vi "FitData.vi"(4 "Fit?":bool=TRUE, 6 "Fmax":dbl format="%#_13g", 7 "Fmin":dbl format="%#_13g", 8 "Yarray":dbl[](array[numeric])) -> (0 "Peak Area (mV-MHz)":dbl=0.0044393014138011675 format="%#_3g", 1 "Center Freq (MHz)":dbl=224.7917277288786, 2 "Amplitude (V)":dbl=0.25549081559976244 format="%#_3g", 3 "NMR Graph + Fit":cluster{cluster{dbl, "Numeric":dbl}[]}[](graph), 5 "# Data points":i32)   [LabVIEW 2018]
uses:
  <vilib>/Analysis/NI_AALPro.lvlib
panel:
  out "Numeric 3":i32
  out "Numeric 2":i32
  out "Yarray 2":dbl[](array[numeric])=[0.01394901666666204, 0.014369016666664246, 0.014784816666666256, 0.015196416666656568, 0.01560381666665861, 0.016007016666660615, 0.015406016666662567, 0.014800816666664496, 0.015191416666666374, 0.015577816666657293, 0.014960016666659214, 0.01533801666666109, 0.014711816666662929, 0.015081416666664724, 0.014446816666666487, 0.014808016666658, 0.014165016666659796, 0.014517816666661555, 0.01386641666666327, 0.014210816666664947, 0.014551016666666583, 0.013887016666658689, 0.013218816666660367, 0.013546416666662002, 0.012869816666663605, 0.013189016666665158, 0.012504016666666673, 0.01181481666665938, 0.01112141666666093, 0.010423816666662443, 0.01072201666666392, 0.011016016666665358, 0.01130581666666675, 0.010591416666660046, 0.009872816666661479, 0.010150016666662872, 0.010423016666664228, 0.010691816666665542, 0.009956416666666822, 0.009216816666660708, 0.009473016666662025, 0.009725016666663297, 0.009972816666664528, 0.00921641666666572, 0.009455816666666873, 0.008691016666661357, 0.00892201666666255, 0.0081488166666637, 0.00837141666666481, 0.009589816666665883, 0.008804016666666914, 0.008014016666661995, 0.008219816666663063, 0.007421416666664099, 0.006618816666665084, 0.0068120166666660355, 0.007001016666666946, 0.007185816666662622, 0.007366416666663572, 0.008542816666664479, 0.009715016666665344, 0.009883016666666175, 0.009046816666666964, 0.010206416666663234, 0.009361816666664066, 0.010513016666664848, 0.010660016666665596, 0.010802816666666305, 0.01094141666666697, 0.012075816666663838, 0.012206016666664543, 0.01233201666666521, 0.013453816666665838, 0.013571416666666423, 0.014684816666666968, 0.015794016666664433, 0.016899016666665018, 0.016999816666665564, 0.01909641666666606, 0.020188816666666526, 0.022277016666666954, 0.025361016666665008, 0.027440816666665473, 0.0305164166666659, 0.03358781666666628, 0.037655016666666624, 0.04171801666666693, 0.04677681666666558, 0.05183141666666592, 0.057881816666666225, 0.06492801666666649, 0.0719700166666667, 0.0800078166666669, 0.08904141666666614, 0.09907081666666637, 0.10909601666666653, 0.1181170166666667, 0.1271338166666668, 0.13414641666666682, 0.14015481666666668, 0.1431590166666668, 0.14415901666666686, 0.14015481666666685, 0.13414641666666682, 0.1261338166666668, 0.11711701666666723, 0.1070960166666672, 0.09807081666666714, 0.08804141666666702, 0.0790078166666669, 0.0709700166666667, 0.06292801666666774, 0.0568818166666676, 0.05083141666666742, 0.04677681666666719, 0.04171801666666693, 0.03665501666666662, 0.03358781666666825, 0.03051641666666799, 0.02744081666666768, 0.026361016666667333, 0.024277016666666956, 0.021188816666666527, 0.018096416666668745, 0.016999816666668367, 0.014899016666667944, 0.012794016666667473, 0.010684816666666971, 0.008571416666669704, 0.00845381666666924, 0.007332016666668731, 0.007206016666668185, 0.006075816666667601, 0.005941416666666973, 0.004802816666670304, 0.0036600166666697145, 0.002513016666669088, 0.0023618166666684176, 0.00220641666666771, 0.0010468166666669637, -0.00011698333332910843, -0.0002849833333298177, -0.0014571833333305688, -0.0016335833333313565, -0.001814183333332187, -0.001998983333333055, -0.002187983333328534, -0.0023811833333293644, -0.0035785833333302364, -0.004780183333331144, -0.005985983333332095, -0.0061959833333330855, -0.006410183333327969, -0.006628583333328922, -0.0068511833333299126, -0.008077983333330947, -0.008308983333332017, -0.008544183333333129, -0.008783583333327419, -0.009027183333328491, -0.009274983333329604, -0.008526983333330757, -0.00878318333333195, -0.010043583333333184, -0.010308183333326877, -0.010576983333328072, -0.011849983333329305, -0.01212718333333058, -0.011408583333331895, -0.01169418333333325, -0.011983983333326348, -0.013277983333327662, -0.01357618333332902, -0.013878583333330414, -0.013185183333331851, -0.013495983333333328, -0.014810983333325829, -0.015130183333327265, -0.015453583333328743, -0.01378118333333026, -0.014112983333331816, -0.015448983333333416, -0.014789183333325323, -0.01513358333332688, -0.01548218333332848, -0.015834983333330117, -0.016191983333331793, -0.016553183333333513, -0.016918583333324827, -0.017288183333326507, -0.017661983333328225, -0.018039983333329984, -0.017422183333331787, -0.018808583333333625, -0.01819918333332434, -0.017593983333326145, -0.016992983333327986, -0.017396183333329866, -0.018803583333331788, -0.019215183333333746, -0.019630983333323873]
  out "Numeric":dbl format="%#_13g"
  out "Linear Slope (V/MHz)":dbl=0.16224074589285484 format="%#_3g"
  out "RMS Fit Error (V)":dbl=0.01168943219151948 format="%#_2g"
  in  "Start sigma (V)":dbl=0.01 format="%#_13g"
  in  "Start offset (V)":dbl format="%#_13g"
  out "FWHM (MHz)":dbl=0.0069336117351933855 format="%#_3g"
  # "Gaussian Fit Results"
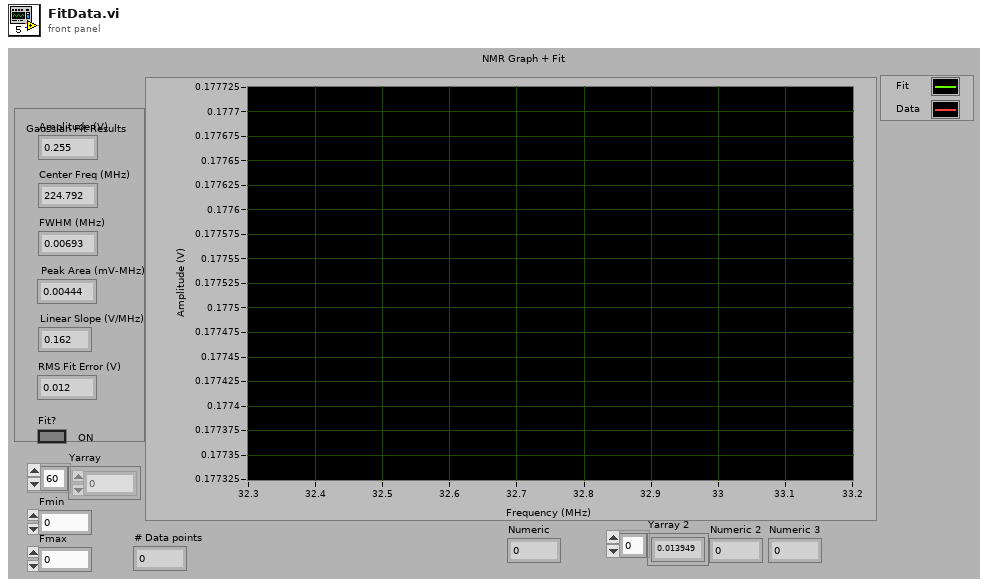
[diagram p1: front panel]
types:
  T1 = cluster{dbl, dbl, "Start sigma (V)":dbl, "Start offset (V)":dbl}
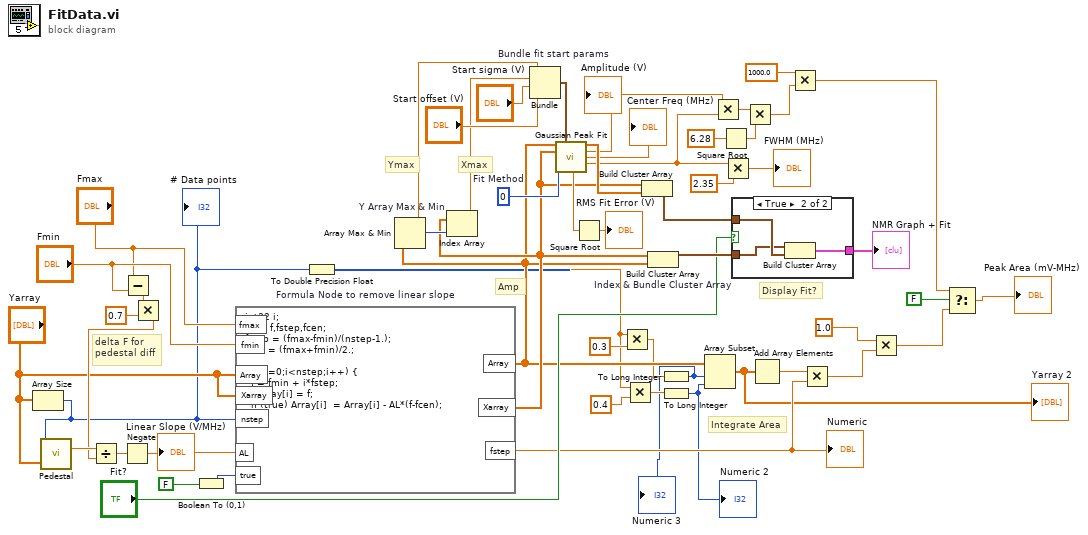
[diagram p0: block diagram]
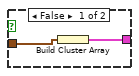
[diagram p2: hidden frame]
diagram:
  w46 = 0  # Fit Method
  # "Integrate Area"
  # "Display Fit?"
  # "Amp"
  # "delta F for\npedestal diff"
  # "Ymax"
  # "Xmax"
  n1 = Array Size(array="Yarray") -> (size(s)=w18:i32)
  "# Data points" <- w18
  n2 = call "Pedestal.vi"("Varray"="Yarray", "ArraySize"=w18) -> ("L-R"=w39:dbl)  [unwired: 1 out]
  n3 = Subtract(x="Fmax", y="Fmin") -> (x-y=w37:dbl)
  n4 = Multiply(x=w37, y=0.7) -> (x*y=w36:dbl)
  n5 = Divide(x=w39, y=w36) -> (x/y=w35:dbl)
  n6 = Negate(x=w35) -> (-x=w34:dbl)
  "Linear Slope (V/MHz)" <- w34
  n7 = Boolean To (0,1)(Boolean=FALSE) -> (0, 1=w23:i16)
  n8 = formula code="int32 i;\nfloat f,fstep,fcen;\nfstep = (fmax-fmin)/(nstep-1.);\nfcen = (fmax+fmin)/2.;\n\nfor (i=0;i<nstep;i++) {\n  f = fmin + i*fstep;\n  Xarray[i] = f;\n  if (true) Array[i]  = Array[i] - AL*(f-fcen);\n}" "Formula Node to remove linear slope"("nstep"=w18, "fmin"="Fmin", "fmax"="Fmax", "AL"=w34, "Array"="Yarray", "Xarray"="Yarray", "true"=w23) -> ("Array"=w19:dbl[], "Xarray"=w27:dbl[], "fstep"=w9:dbl)
  "Numeric" <- w9
  n9 = To Double Precision Float(number=w18) -> (double precision float=w5:dbl)
  n10 = Array Max & Min "Y Array Max & Min"(array=w19) -> (max value=w45:dbl, max index (indices)=w44:i32)  [unwired: 2 out]
  n11 = Index Array "Index Array"(array=w27, index=w44) -> (element=w31:dbl)
  n12 = Bundle "Bundle fit start params"(w45, w31, "Start sigma (V)"="Start sigma (V)", "Start offset (V)"="Start offset (V)") -> (w51:T1)  [unwired: 1 in]
  n13 = call <vilib>:"Gaussian Peak Fit.vi"("Y"=w19, "initial guess"=w51, "X"=w27, "method"=w46) -> ("Best Gaussian Fit"=w54:dbl[], "amplitude"=w43:dbl, "center"=→"Center Freq (MHz)":dbl, "standard deviation"=w30:dbl, "residue"=w33:dbl)  [unwired: 5 in, 2 out]
  "Amplitude (V)" <- w43
  n14 = Square Root(x=w33) -> (sqrt(x)=→"RMS Fit Error (V)":dbl)
  n15 = Multiply(x=w5, y=0.3) -> (x*y=w15:dbl)
  n16 = Multiply(x=w5, y=0.4) -> (x*y=w14:dbl)
  n17 = Build Cluster Array ("Index & Bundle Cluster Array")(w27, w54) -> (w50:cluster{dbl, "Numeric":dbl}[])
  n18 = Build Cluster Array "Index & Bundle Cluster Array"(w27, w19) -> (w49:cluster{dbl, dbl}[])
  n19 = To Long Integer(number=w15) -> (32bit integer=w6:i32)
  "Numeric 3" <- w6
  n20 = To Long Integer(number=w14) -> (32bit integer=w7:i32)
  "Numeric 2" <- w7
  n21 = Array Subset "Array Subset"(array=w19, index=w6, length=w7) -> (w8:dbl[])
  "Yarray 2" <- w8
  n22 = Multiply(x=w43, y=w30) -> (x*y=w40:dbl)
  n23 = Square Root(x=6.28) -> (sqrt(x)=w41:dbl)
  n24 = Multiply(x=w30, y=2.35) -> (x*y=→"FWHM (MHz)":dbl)
  n25 = case shown="True" "Fit?" {
    tunnel: w50 -> [_ w58]
    tunnel: w49 -> [w56 w57]
    tunnel: [w55 w59] -> w48
    frame False {
      n26 = Build Cluster Array "Build Cluster Array"(w56) -> (w55:cluster{cluster{dbl, dbl}[]}[])
    }
    frame True {
      n27 = Build Cluster Array "Build Cluster Array"(w57, w58) -> (w59:cluster{cluster{dbl, "Numeric":dbl}[]}[])
    }
  }
  "NMR Graph + Fit" <- w48
  n28 = Multiply(x=w40, y=w41) -> (x*y=w21:dbl)
  n29 = Add Array Elements(numeric array=w8) -> (sum=w13:dbl)
  n30 = Multiply(x=1000.0, y=w21) -> (x*y=w12:dbl)
  n31 = Multiply(x=w13, y=w9) -> (x*y=w4:dbl)
  n32 = Multiply(x=1.0, y=w4) -> (x*y=w2:dbl)
  n33 = Select(t=w12, s=FALSE, f=w2) -> (s? t:f=→"Peak Area (mV-MHz)":dbl)
